vi "Power Fit (LS).vi"(0 "Y":dbl[](array[numeric]), 5 "X":dbl[](array[numeric]), 7 "Weight":dbl[](array[numeric]), 9 "tolerance":dbl=0.0001 format="%#_3g", 11 "Initial Coefficients":dbl[](array[numeric])) -> (4 "Best Power Fit":dbl[](array[numeric]), 6 "amplitude":dbl, 8 "power":dbl, 14 "residue":dbl, 15 "error":i32)   [LabVIEW 2017, in "NI_AALPro.lvlib"]
uses:
  <vilib>/Analysis/NI_AALPro.lvlib
  <resource>/lvanlys.dll
panel:
  # "LS Power Fit"
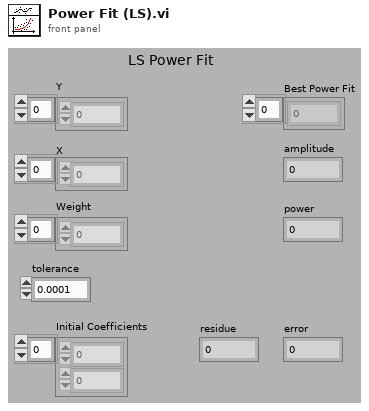
[diagram p1: front panel]
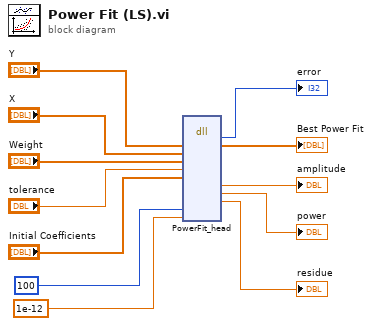
[diagram p0: block diagram]
diagram:
  n1 = dll-call lib="e:/builds/penguin/labview/branches/2017/dev/dist/resource/lvanlys.*" fn="PowerFit_head"("y"="Y", "x"="X", "weight"="Weight", "tolerance"="tolerance", "initialCoef"="Initial Coefficients", "maxIter"=100, "absTol"=1e-12) -> (→"error":i32, "y"=→"Best Power Fit":dbl[], "amplitude"=→"amplitude":dbl, "power"=→"power":dbl, "mse"=→"residue":dbl)  [unwired: 12 in, 2 out]
